vi "GPIB_meas_resistance_over_Time.vi"() -> ()   [LabVIEW 2021]
uses:
  <vilib>/Utility/miscctls.llb/LVRectTypeDef.ctl
  <vilib>/UPVI/lvhdf5/group.llb/H5G_obj_t.ctl
  <vilib>/UPVI/lvhdf5/dataset.llb/LVH5D Operation.ctl
  <instrlib>/Agilent 34401/Public/Data/Read (Single Point).vi
  <vilib>/UPVI/lvhdf5/utility.llb/Select HDF5 Dialog.vi
  <vilib>/UPVI/lvhdf5/utility.llb/Select HDF5 Dialog (Object Only).vi
  <vilib>/UPVI/lvhdf5/dataset.llb/Simple H5Dwrite (Variant).vi
  <vilib>/UPVI/lvhdf5/dataset.llb/Simple H5Dwrite.xnode
  <vilib>/UPVI/lvhdf5/library.llb/HDF5 Ref.ctl
  <instrlib>/Agilent 34401/Agilent 34401.lvlib
  <vilib>/UPVI/lvhdf5/library.llb/HDF5 Ref.lvclass
  <vilib>/UPVI/lvhdf5/identifier.llb/Not an HDF5 Refnum Constant.vi
  <vilib>/Utility/error.llb/Error Cluster From Error Code.vi
  <vilib>/UPVI/lvhdf5/dataset.llb/OpenCreateReplace Dataset by Element Type.vi
  <vilib>/UPVI/lvhdf5/dataspace.llb/H5Sselect_hyperslab.vi
  <vilib>/UPVI/lvhdf5/dataset.llb/H5Dwrite (Variant).vi
  <vilib>/UPVI/lvhdf5/dataset.llb/H5Dget_space.vi
  <vilib>/UPVI/lvhdf5/attribute.llb/private/LVH5AwriteWDTAttrs.vi
  <vilib>/UPVI/lvhdf5/dataspace.llb/H5Sclose.vi
  <vilib>/UPVI/lvhdf5/dataset.llb/H5Dclose.vi
  <vilib>/UPVI/lvhdf5/file.llb/OpenCreateReplace HDF5 File.vi
  <vilib>/UPVI/lvhdf5/file.llb/LVH5F Operation.ctl
  <vilib>/UPVI/lvhdf5/utility.llb/Select HDF5 Dialog (File and Object).vi
panel:
  out "Temp 5: Water tank Small":dbl
  out "Numeric":i32
  out "Temperatures":dbl[][](graph)=[[26.058823529411768, 26.058823529411768, 26.058823529411768, 26.058823529411768, 26.058823529411768, 26.058823529411768, 26.058823529411768, 26.058823529411768, 26.058823529411768, 26.058823529411768, 26.058823529411768, 26.058823529411768, 26.058823529411768, 26.058823529411768, 26.058823529411768, 26.058823529411768, 26.058823529411768, 26.058823529411768, 26.058823529411768, 26.058823529411768, 26.058823529411768, 26.058823529411768, 26.058823529411768, 26.058823529411768, 26.058823529411768, 26.058823529411768, 26.058823529411768, 26.058823529411768, 26.058823529411768, 26.058823529411768, 26.058823529411768, 26.058823529411768, 26.058823529411768, 26.058823529411768, 26.058823529411768, 26.058823529411768, 26.058823529411768, 26.058823529411768, 26.058823529411768, 26.058823529411768, 26.058823529411768, 26.058823529411768, 26.058823529411768, 26.058823529411768, 26.058823529411768, 26.058823529411768, 26.058823529411768, 26.058823529411768, 26.058823529411768, 26.058823529411768, 26.058823529411768, 26.058823529411768, 26.058823529411768, 26.058823529411768, 26.058823529411768, 26.058823529411768, 26.058823529411768, 26.058823529411768, 26.058823529411768, 26.058823529411768, 26.058823529411768, 26.058823529411768, 26.058823529411768, 26.058823529411768, 26.058823529411768, 26.058823529411768, 26.058823529411768, 26.058823529411768, 26.058823529411768, 26.058823529411768, 26.058823529411768, 26.058823529411768, 26.058823529411768, 26.058823529411768, 26.058823529411768, 26.058823529411768, 26.058823529411768, 26.058823529411768, 26.058823529411768, 26.058823529411768, 26.058823529411768, 26.058823529411768, 26.058823529411768, 26.058823529411768, 26.058823529411768, 26.058823529411768, 26.058823529411768, 26.058823529411768, 26.058823529411768, 26.058823529411768, 26.058823529411768, 26.058823529411768, 26.058823529411768, 26.058823529411768, 26.058823529411768, 26.058823529411768, 26.058823529411768, 26.058823529411768, 26.058823529411768, 26.058823529411768, 26.058823529411768, 26.058823529411768, 26.058823529411768], [26.058823529411768, 26.058823529411768, 26.058823529411768, 26.058823529411768, 26.058823529411768, 26.058823529411768, 26.058823529411768, 26.058823529411768, 26.058823529411768, 26.058823529411768, 26.058823529411768, 26.058823529411768, 26.058823529411768, 26.058823529411768, 26.058823529411768, 26.058823529411768, 26.058823529411768, 26.058823529411768, 26.058823529411768, 26.058823529411768, 26.058823529411768, 26.058823529411768, 26.058823529411768, 26.058823529411768, 26.058823529411768, 26.058823529411768, 26.058823529411768, 26.058823529411768, 26.058823529411768, 26.058823529411768, 26.058823529411768, 26.058823529411768, 26.058823529411768, 26.058823529411768, 26.058823529411768, 26.058823529411768, 26.058823529411768, 26.058823529411768, 26.058823529411768, 26.058823529411768, 26.058823529411768, 26.058823529411768, 26.058823529411768, 26.058823529411768, 26.058823529411768, 26.058823529411768, 26.058823529411768, 26.058823529411768, 26.058823529411768, 26.058823529411768, 26.058823529411768, 26.058823529411768, 26.058823529411768, 26.058823529411768, 26.058823529411768, 26.058823529411768, 26.058823529411768, 26.058823529411768, 26.058823529411768, 26.058823529411768, 26.058823529411768, 26.058823529411768, 26.058823529411768, 26.058823529411768, 26.058823529411768, 26.058823529411768, 26.058823529411768, 26.058823529411768, 26.058823529411768, 26.058823529411768, 26.058823529411768, 26.058823529411768, 26.058823529411768, 26.058823529411768, 26.058823529411768, 26.058823529411768, 26.058823529411768, 26.058823529411768, 26.058823529411768, 26.058823529411768, 26.058823529411768, 26.058823529411768, 26.058823529411768, 26.058823529411768, 26.058823529411768, 26.058823529411768, 26.058823529411768, 26.058823529411768, 26.058823529411768, 26.058823529411768, 26.058823529411768, 26.058823529411768, 26.058823529411768, 26.058823529411768, 26.058823529411768, 26.058823529411768, 26.058823529411768, 26.058823529411768, 26.058823529411768, 26.058823529411768, 26.058823529411768, 26.058823529411768, 26.058823529411768], [24.501960784313724, 24.501960784313724, 24.501960784313724, 24.501960784313724, 24.501960784313724, 24.501960784313724, 24.501960784313724, 24.501960784313724, 24.501960784313724, 24.501960784313724, 24.501960784313724, 24.501960784313724, 24.501960784313724, 24.847058823529412, 24.501960784313724, 24.501960784313724, 24.501960784313724, 24.501960784313724, 24.501960784313724, 24.847058823529412, 24.847058823529412, 24.847058823529412, 24.847058823529412, 24.847058823529412, 24.847058823529412, 24.847058823529412, 24.847058823529412, 24.847058823529412, 24.847058823529412, 24.847058823529412, 24.847058823529412, 24.847058823529412, 24.847058823529412, 24.847058823529412, 24.847058823529412, 24.847058823529412, 24.847058823529412, 24.847058823529412, 24.847058823529412, 24.847058823529412, 24.847058823529412, 24.847058823529412, 24.847058823529412, 24.847058823529412, 24.847058823529412, 24.847058823529412, 24.847058823529412, 24.847058823529412, 24.847058823529412, 24.847058823529412, 24.847058823529412, 24.847058823529412, 24.847058823529412, 24.847058823529412, 24.847058823529412, 24.847058823529412, 24.847058823529412, 24.847058823529412, 24.847058823529412, 24.847058823529412, 24.847058823529412, 24.847058823529412, 24.847058823529412, 24.847058823529412, 24.847058823529412, 24.847058823529412, 24.847058823529412, 24.847058823529412, 24.847058823529412, 24.847058823529412, 24.847058823529412, 24.847058823529412, 24.847058823529412, 25.192156862745097, 25.192156862745097, 25.192156862745097, 25.192156862745097, 25.192156862745097, 25.192156862745097, 25.192156862745097, 25.192156862745097, 25.192156862745097, 25.192156862745097, 25.192156862745097, 25.192156862745097, 25.192156862745097, 25.192156862745097, 25.192156862745097, 25.192156862745097, 25.192156862745097, 25.192156862745097, 25.192156862745097, 25.192156862745097, 25.192156862745097, 25.192156862745097, 25.192156862745097, 25.192156862745097, 25.192156862745097, 25.192156862745097, 25.192156862745097, 25.192156862745097, 25.192156862745097, 25.192156862745097], [24.15686274509804, 24.15686274509804, 24.15686274509804, 24.15686274509804, 24.15686274509804, 24.15686274509804, 24.15686274509804, 24.15686274509804, 24.15686274509804, 24.15686274509804, 24.15686274509804, 24.15686274509804, 24.15686274509804, 24.15686274509804, 24.15686274509804, 24.15686274509804, 24.15686274509804, 24.15686274509804, 24.15686274509804, 24.15686274509804, 24.15686274509804, 24.15686274509804, 24.15686274509804, 24.15686274509804, 24.15686274509804, 24.15686274509804, 24.15686274509804, 24.15686274509804, 24.15686274509804, 24.15686274509804, 24.15686274509804, 24.15686274509804, 24.15686274509804, 24.15686274509804, 24.15686274509804, 24.15686274509804, 24.15686274509804, 24.15686274509804, 24.15686274509804, 24.15686274509804, 24.15686274509804, 24.15686274509804, 24.15686274509804, 24.15686274509804, 24.15686274509804, 24.15686274509804, 24.15686274509804, 24.15686274509804, 24.15686274509804, 24.15686274509804, 24.15686274509804, 24.15686274509804, 24.15686274509804, 24.15686274509804, 24.15686274509804, 24.15686274509804, 24.15686274509804, 24.15686274509804, 24.15686274509804, 24.15686274509804, 24.15686274509804, 24.15686274509804, 24.15686274509804, 24.15686274509804, 24.15686274509804, 24.15686274509804, 24.15686274509804, 24.15686274509804, 24.15686274509804, 24.15686274509804, 24.15686274509804, 24.15686274509804, 24.15686274509804, 24.15686274509804, 24.15686274509804, 24.501960784313724, 24.501960784313724, 24.501960784313724, 24.501960784313724, 24.501960784313724, 24.501960784313724, 24.501960784313724, 24.501960784313724, 24.501960784313724, 24.501960784313724, 24.501960784313724, 24.501960784313724, 24.501960784313724, 24.501960784313724, 24.501960784313724, 24.501960784313724, 24.501960784313724, 24.501960784313724, 24.501960784313724, 24.501960784313724, 24.501960784313724, 24.501960784313724, 24.501960784313724, 24.501960784313724, 24.501960784313724, 24.501960784313724, 24.501960784313724, 24.501960784313724]]
  out "Temp 4: Water tank Big":dbl=24.501960784313724
  out "Temp 3: Tx Filt Xfmer":dbl=25.192156862745097
  out "Temp 2: Tx Filt L6":dbl=26.058823529411768
  out "Temp 1: Tx Filt L7":dbl=26.058823529411768
  out "Saved as:":string
  in  "Save?":bool
  in  "in:":path=path "D:/MPIdata"
  in  "desc":string
  out "temp":dbl
  in  "stop":bool
  out "Waveform Graph":dbl[](graph)
  out "raw measurement":dbl
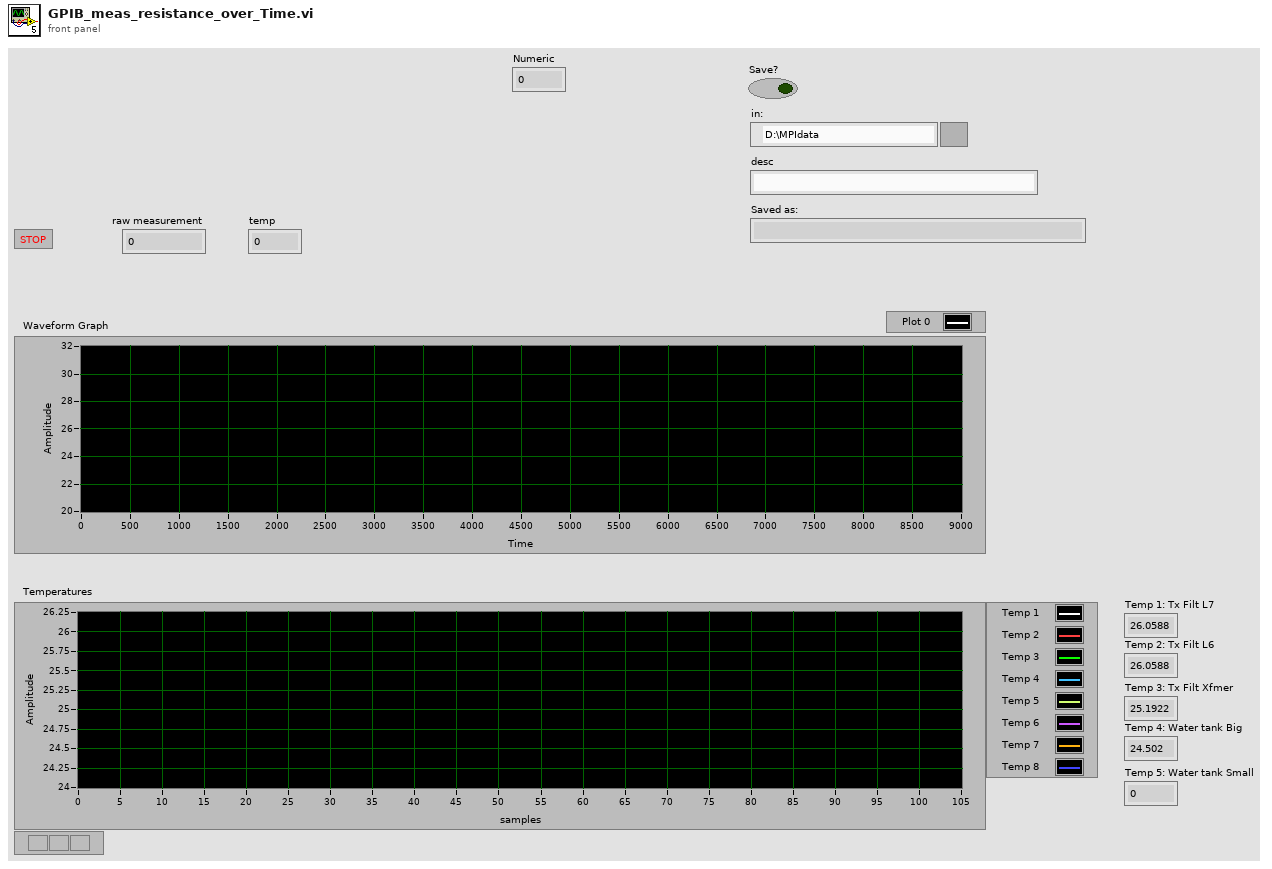
[diagram p1: front panel]
types:
  T1 = typedef "LVRectTypeDef.ctl" = cluster{"Left":i16, "Top":i16, "Right":i16, "Bottom":i16}
  T2 = cluster{"Behavior":enum32{"Invalid", "Default", "Floating", "Floating/Auto-Hide", "Modal"}, "Position":T1, "Center":bool, "Title":string}
  T3 = typedef "LVH5F Operation.ctl" = enum16{"open", "open or create", "create or replace", "create or replace (with confirmation)", "create", "open (read only)"}
  T4 = typedef "LVH5D Operation.ctl" = enum16{"open", "replace", "create", "open or create", "create or replace", "create or replace with confirmation"}
  T5 = typedef "H5G_obj_t.ctl" = i32
  T6 = cluster{"Object Types (any)":T5[], "Object Pattern":string}
  T7 = typedef "HDF5 Ref.ctl" = refnum<class "HDF5 Ref.lvclass">
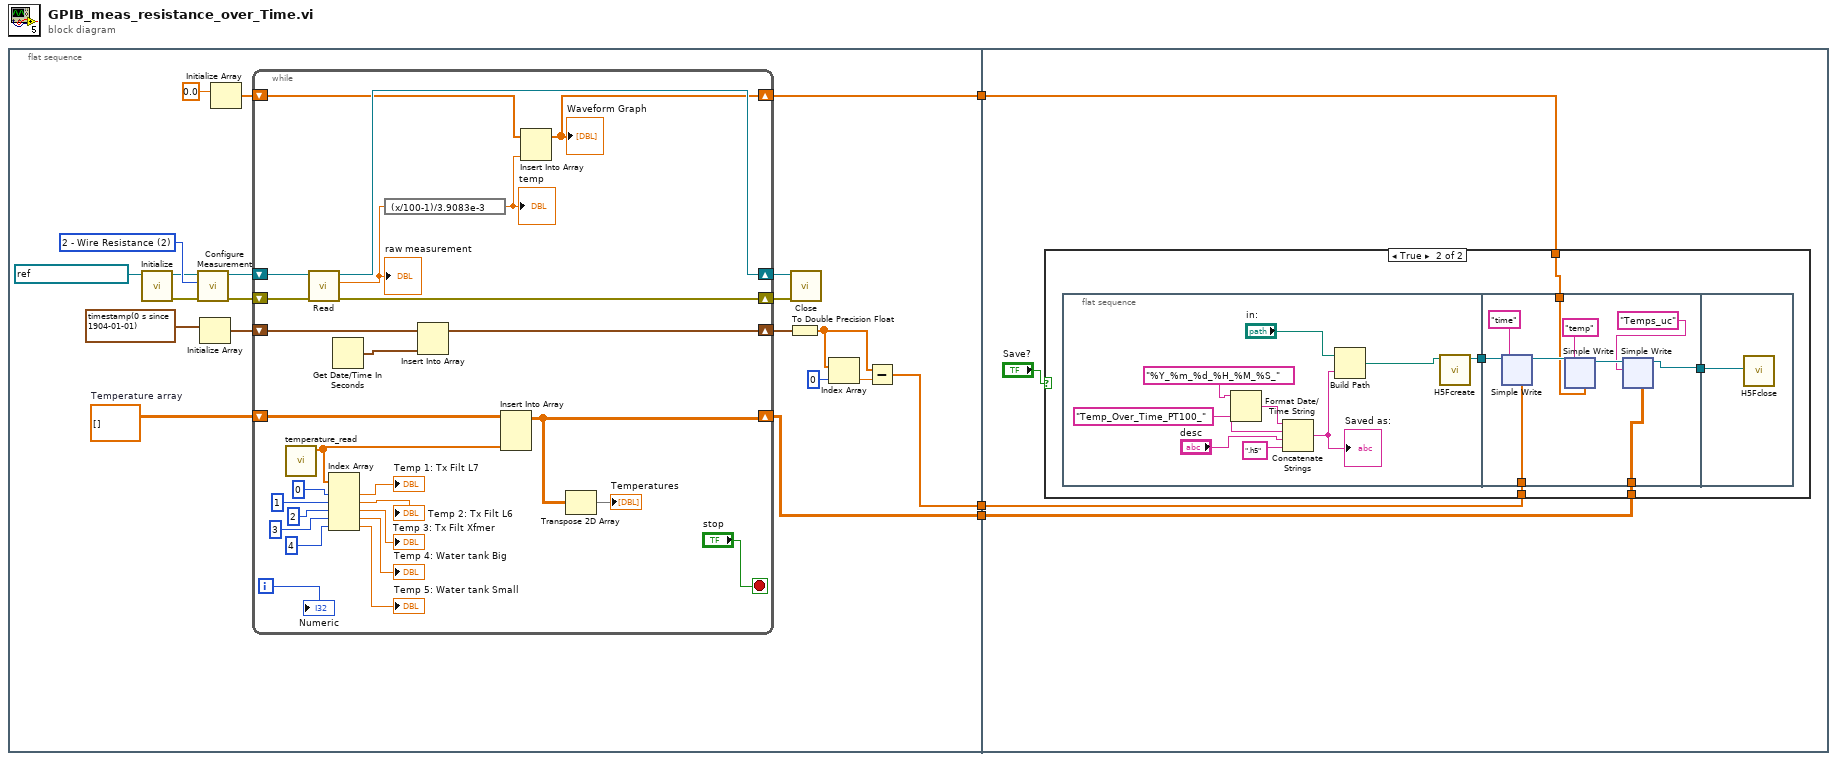
[diagram p0: block diagram]
diagram:
  n1 = flat-sequence {
    tunnel: [w11] -> w3
    tunnel: [w6] -> w2
    tunnel: [w4] -> w1
    tunnel: w3 -> [w53]
    tunnel: w2 -> [w52]
    tunnel: w1 -> [w51]
    frame #0 {
      w5 = dbl[][] []  # Temperature array
      w20 = u16 2 items=["DC Voltage", "AC Voltage", "2 - Wire Resistance", "4 - Wire Resistance", "DC Current", "AC Current", "Frequency", "Period", "Continuity", "Diode Checking", "VDC:VDC Ratio", "Temperature", "Capacitance"] ("Function (0: DC Voltage)")
      n2 = call <instrlib>:"Initialize.vi"("VISA resource name"=refnum<visa-resource-name> "GPIB0::22::INSTR") -> ("error out"=w18:errorcluster, "VISA resource name out"=w19:refnum<visa-resource-name>)  [unwired: 9 in]
      n3 = call <instrlib>:"Configure Measurement.vi"("error in (no error)"=w18, "Function (0: DC Voltage)"=w20, "VISA resource name"=w19) -> ("error out"=w17:errorcluster, "VISA resource name out"=w16:refnum<visa-resource-name>)  [unwired: 7 in]
      n4 = Initialize Array(timestamp(0 s since 1904-01-01) ("current time")) -> (w12:timestamp[])  [unwired: 1 in]
      n5 = Initialize Array(0.0 ("element")) -> (w15:dbl[])  [unwired: 1 in]
      n6 = while {
        shift-right: [w49] -> w21
        shift-left: w17 -> [w48]
        shift-right: [w50] -> w22
        shift-left: w16 -> [w47]
        shift-right: [w41] -> w11
        shift-left: w15 -> [w46]
        shift-right: [w42] -> w10
        shift-left: w12 -> [w44]
        shift-right: [w26] -> w4
        shift-left: w5 -> [w27]
        i -> [w38]
        stop <- "stop" stop-if-true
        n7 = call "temperature_read.vi"() -> ("temperature array"=w29:dbl[])  [unwired: 10 in]
        n8 = call-poly <instrlib>:"Read.vi"("error in (no error)"=w48, "VISA resource name"=w47) -> ("error out"=w49:errorcluster, "Measurement"=w40:dbl, "VISA resource name out"=w50:refnum<visa-resource-name>)  [unwired: 7 in]
        "raw measurement" <- w40
        n9 = Index Array(array=w29, index #1=0 ("index"), index #2=1 ("index"), index #3=2 ("index"), index #4=3 ("index"), index #5=4 ("index")) -> (element #1=→"Temp 1: Tx Filt L7":dbl, element #2=→"Temp 2: Tx Filt L6":dbl, element #3=→"Temp 3: Tx Filt Xfmer":dbl, element #4=→"Temp 4: Water tank Big":dbl, element #5=→"Temp 5: Water tank Small":dbl)
        n10 = Get Date/Time In Seconds() -> (seconds since 1Jan1904=w43:timestamp)
        n11 = expression code="(x/100-1)/3.9083e-3"(w40) -> (w39:dbl)
        "temp" <- w39
        n12 = Insert Into Array(array=w44, new element=w43) -> (w42:timestamp[])  [unwired: 1 in]
        n13 = Insert Into Array(array=w27, new element=w29) -> (w26:dbl[][])  [unwired: 2 in]
        n14 = Insert Into Array(array=w46, new element=w39) -> (w41:dbl[])  [unwired: 1 in]
        "Waveform Graph" <- w41
        n15 = Transpose 2D Array(2D array=w26) -> (transposed array=→"Temperatures":dbl[][])
        "Numeric" <- w38
      }
      n16 = To Double Precision Float(number=w10) -> (double precision float=w8:dbl[])
      n17 = call <instrlib>:"Close.vi"("error in (no error)"=w21, "VISA resource name"=w22) -> ()  [unwired: 9 in, 1 out]
      n18 = Index Array(array=w8, index=0) -> (element=w9:dbl)
      n19 = Subtract(x=w8, y=w9) -> (x-y=w6:dbl[])
    }
    frame #1 {
      n20 = case shown="True" "Save?" {
        tunnel: w53 -> [_ w57]
        tunnel: w52 -> [_ w56]
        tunnel: w51 -> [_ w55]
        frame False {
        }
        frame True {
          n21 = flat-sequence {
            tunnel: [w63] -> w59
            tunnel: w59 -> [w78]
            tunnel: [w71] -> w58
            tunnel: w57 -> [w75]
            tunnel: w56 -> [w73]
            tunnel: w55 -> [w69]
            tunnel: w58 -> [w685]
            frame #0 {
              n22 = Format Date/Time String(time format string (%c)="%Y_%m_%d_%H_%M_%S_") -> (date/time string=w67:string)  [unwired: 2 in]
              n23 = Concatenate Strings(w67, "Temp_Over_Time_PT100_" ("string"), "desc", ".h5" ("string")) -> (w65:string)
              "Saved as:" <- w65
              n24 = Build Path(base path="in:", name or relative path=w65) -> (appended path=w64:path)
              n25 = call <vilib>:"H5Fcreate.vi"("path"=w64) -> ("HDF5 Ref"=w63:T7)  [unwired: 7 in, 1 out]
            }
            frame #1 {
              n26 = xnode "Simple Write"("Dataset Path"="time", "HDF5 Path or Ref"=w78, "Data"=w73) -> ("HDF5 Ref out"=w76:T7)  [unwired: 5 in, 2 out]
              n27 = xnode "Simple Write"("Dataset Path"="temp", "HDF5 Path or Ref"=w76, "Data"=w75) -> ("HDF5 Ref out"=w72:T7)  [unwired: 5 in, 2 out]
              n28 = xnode "Simple Write"("Dataset Path"="Temps_uc", "HDF5 Path or Ref"=w72, "Data"=w69) -> ("HDF5 Ref out"=w71:T7)  [unwired: 5 in, 2 out]
            }
            frame #2 {
              n29 = call <vilib>:"H5Fclose.vi"("HDF5 Ref"=w685) -> ()  [unwired: 8 in, 1 out]
            }
          }
        }
      }
    }
  }
